vi "Load Configuration.vi"(8 "error in":errorcluster, 11 "Configuration UI in":refnum<class "Configuration UI.lvclass">) -> (0 "error out":errorcluster, 3 "Configuration UI out":refnum<class "Configuration UI.lvclass">)   [LabVIEW 2019, in "Configuration UI.lvlib" / "Configuration UI.lvclass"]
doc: "This routine loads the config.ini file to memory, guaranteeing that at the start of the program the GUI matches the config.ini values."
uses:
  Project/Configuration UI.lvclass
  C:/Users/Public/Documents/Development/builds/Engine/Engine.lvlibp/Project/Engine.lvclass
  Project/Configuration UI.lvclass/Configuration UI.ctl
  Accessors/Read Instrument Listbox.vi
  Accessors/Read Config.vi
  Accessors/Write Instrument Listbox.vi
  Accessors/Write Config.vi
  builds/Engine/Engine.lvlibp/Accessors/Read Directory.vi
  builds/Tools/Config.lvlibp/Accessors/Read Device List.vi
  builds/Tools/Config.lvlibp/Config.lvclass
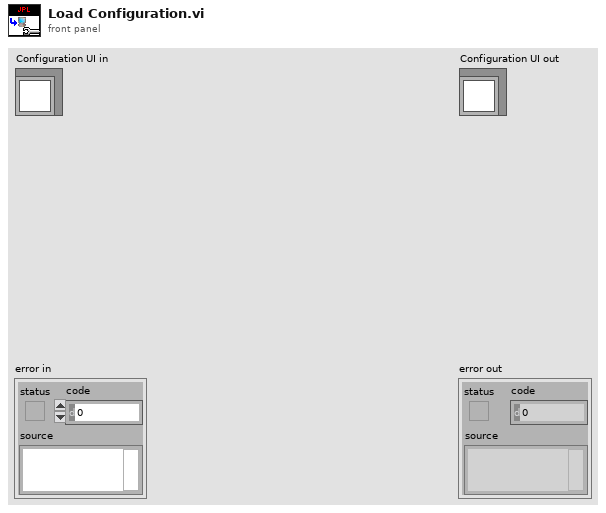
[diagram p1: front panel]
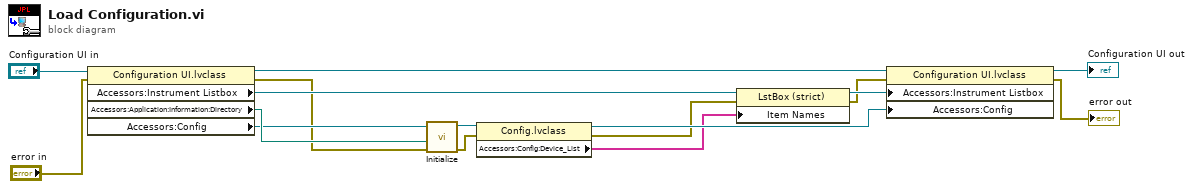
[diagram p0: block diagram]
diagram:
  n1 = property class="Configuration UI.lvclass"(reference="Configuration UI in", error in="error in") -> (reference out=w15:refnum<class "Configuration UI.lvclass">, error out=w9:errorcluster, "Accessors:Instrument Listbox"=w13:refnum<vi>, "Accessors:Application:Information:Directory"=w11:path, "Accessors:Config"=w10:refnum<class "Config.lvclass">)
  n2 = call-dynamic "Initialize.vi"("error in"=w9, "Path"=w11, "Config in"=w10) -> ("error out"=w4:errorcluster, "Config out"=w7:refnum<class "Config.lvclass">)  [unwired: 7 in]
  n3 = property class="Config.lvclass"(reference=w7, error in=w4) -> (reference out=w6:refnum<class "Config.lvclass">, error out=w3:errorcluster, "Accessors:Config:Device_List"=w1:string[])
  n4 = property class="LstBox (strict)"(reference=w13, error in=w3, "Item Names"=w1) -> (reference out=w12:refnum<vi>, error out=w2:errorcluster)
  n5 = property class="Configuration UI.lvclass"(reference=w15, error in=w2, "Accessors:Instrument Listbox"=w12, "Accessors:Config"=w6) -> (reference out=→"Configuration UI out":refnum<class "Configuration UI.lvclass">, error out=→"error out":errorcluster)
